vi "SetReportPath.vi"(8 "error in (no error)":errorcluster, 11 "default path":path) -> (0 "error out":errorcluster, 3 "ResultPath":path)   [LabVIEW 2014]
uses:
  <vilib>/Utility/config.llb/Write Key (Path).vi
  <vilib>/Utility/config.llb/NI_LVConfig.lvlib
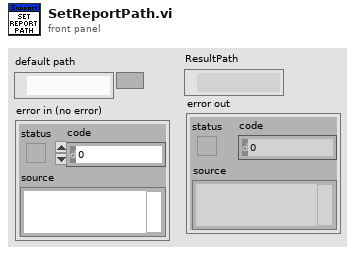
[diagram p1: front panel]
types:
  T1 = typedef "NI_LVConfig.lvlib/Config Data RefNum.ctl" = refnum<k1>
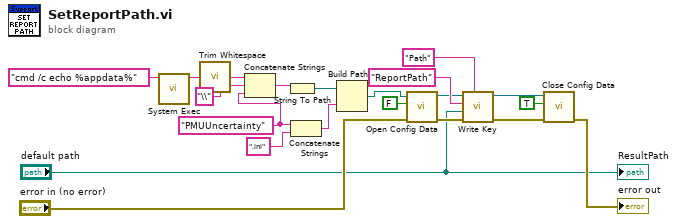
[diagram p0: block diagram]
diagram:
  w18 = "PMUUncertainty" ("string")
  n1 = call <vilib>:"System Exec.vi"("command line"="cmd /c echo %appdata%") -> ("standard output"=w14:string)  [unwired: 7 in, 3 out]
  n2 = call <vilib>:"Trim Whitespace.vi"("string"=w14) -> ("trimmed string"=w13:string)  [unwired: 1 in]
  n3 = Concatenate Strings(w13, "\\" ("string"), w18) -> (w20:string)
  n4 = String To Path(string=w20) -> (path=w19:path)
  n5 = Concatenate Strings(w18, ".ini" ("string")) -> (w16:string)
  n6 = Build Path(base path=w19, name or relative path=w16) -> (appended path=w11:path)
  n7 = call <vilib>:"Open Config Data.vi"("error in (no error)"="error in (no error)", "create file if necessary (T)"=FALSE, "configuration file path"=w11) -> ("error out"=w9:errorcluster, "refnum"=w6:T1)  [unwired: 6 in, 1 out]
  n8 = call-poly <vilib>:"Write Key.vi"("section"="Path", "error in (no error)"=w9, "value"="default path", "key"="ReportPath", "refnum"=w6) -> ("error out"=w3:errorcluster, "refnum out"=w5:T1)  [unwired: 4 in, 1 out]
  n9 = call <vilib>:"Close Config Data.vi"("error in (no error)"=w3, "write file if changed (T)"=TRUE, "refnum"=w5) -> ("error out"=→"error out":errorcluster)  [unwired: 7 in, 1 out]
  "ResultPath" <- "default path"
